vi "Read configuration.vi"(8 "error in":errorcluster, 11 "cfg cRIO root in":refnum<class "cRIO  node root.lvclass">) -> (0 "error out":errorcluster, 2 "configuration":refnum<class "NISE_CEF_serializable configuration.lvclass">, 3 "cfg cRIO root out":refnum<class "cRIO  node root.lvclass">)   [LabVIEW 2013, in "cRIO  node root.lvclass"]
uses:
  cRIO  node root.lvclass
  CEF_TreeControl/serializable configuration/NISE_CEF_serializable configuration.lvclass
  cRIO  node root.lvclass/cRIO  node root.ctl
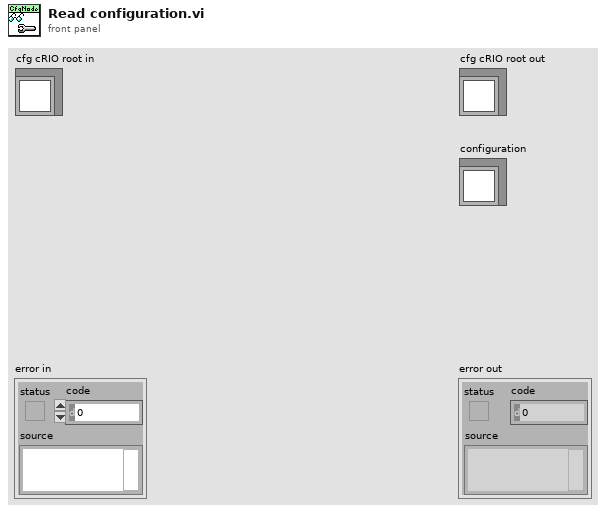
[diagram p1: front panel]
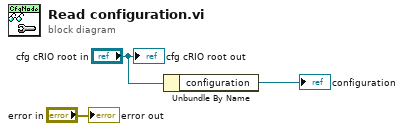
[diagram p0: block diagram]
diagram:
  n1 = Unbundle By Name("cfg cRIO root in") -> ("configuration"=→"configuration":refnum<class "cRIO configuration.lvclass">)
  "error out" <- "error in"
  "cfg cRIO root out" <- "cfg cRIO root in"
